vi "Mod_OFDM_Complex_Symbols _Generation.vi"(0 "Configuration in":variant, 11 "error in (no error)":errorcluster) -> (2 "Bits Generated":i8[](array[numeric]), 4 "Complex Symbols w/ Cyclic prefix":cdb[](array[numeric]), 6 "Parameters per Ofdm Symbol":T1 {"Data Source"."Data Source"."Register Initial State" format="%08x"}, 8 "Complex Symbols":cdb[][](array[numeric]), 10 "Pulse Shaping Parameters":T2={"System Filter"={"TX Filter"=enum."Root Raised Cos", "Alpha"=0.5, "filter length"=8}, "Modulation system parameters"={"samples per symbol (16)"=16}, "symbol rate (Hz)"=1.0} {"symbol rate (Hz)" min=1.0 step=1.0 format="%.2p"; "Modulation system parameters"."samples per symbol (16)" step=2; "System Filter"."Alpha" min=0.0 max=1.0 step=0.05 format="%.2f"}, 13 "Complex Mapping":cdb[][](array[numeric]), 15 "error out":errorcluster)   [LabVIEW 2010]
doc: "The VI generates the baseband complex symbols for the configured OFDM frame. Following five functions are performed by VI.l\n\n1. Converts Variant: Recovers the configuration settings from the variant into an array of clusters. The size of the array is the number of OFDM Symbols in the frame. Each cluster contains the configuration settings pertaining to a specific OFDM symbol. \n\n2. Generates Bits: For each OFDM Symbol in the Frame bits are generated depending on the data sources assigned to the sub carriers and the configuration settings of the data sources.\n\n3. Performs Complex Mapping: Complex Mapping of the bits generated are performed based on the modulation scheme selected.\n\n4. Applies IFFT: Block IFFT is performed on the complex signal\n\nNote: The common way to implement the inverse Fourier transform is by an inverse Fast Fourier Transform (IFFT). If, for example, a 64-point IFFT is used, the coefficients 0 to +31 are mapped to the same numbered IFFT inputs, while the coefficients -32 to -1 are copied into IFFT inputs +32 to +63. \n\n5. After performing an IFFT, the output is cyclically extended to the desired length by prepending the output of the IFFT."
uses:
  Controls(Type_DEf)/Configure Pulse Shaping.ctl
  Controls(Type_DEf)/Parameters per Ofdm Symbol.ctl
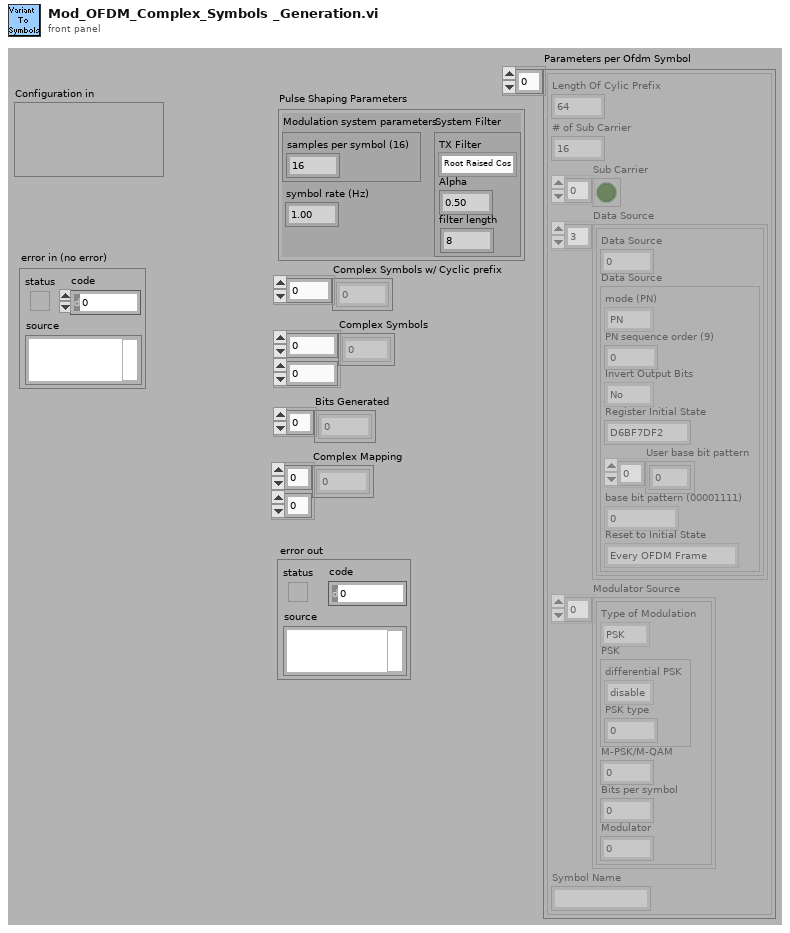
[diagram p1: front panel]
types:
  T1 = typedef "Parameters per Ofdm Symbol.ctl" = cluster{"Length Of Cylic Prefix":i32, "# of Sub Carrier":i32, "Sub Carrier":bool[], "Data Source":cluster{"Data Source":u16, "Data Source":cluster{"mode (PN)":enum16{"PN", "pattern", "user"}, "PN sequence order (9)":i32, "Invert Output Bits":enum16{"No", "Yes"}, "Register Initial State":u32, "User base bit pattern":i8[], "base bit pattern (00001111)":enum16{"0", "1", "01", "0011", "00001111"}, "Reset to Initial State":enum16{"Every OFDM Frame", "Every OFDM Symbol", "Every Sub Carrier"}}}[], "Modulator Source":cluster{"Type of Modulation":enum16{"PSK", "QAM"}, "PSK":cluster{"differential PSK":enum16{"disable", "enable"}, "PSK type":u16}, "M-PSK/M-QAM":i32, "Bits per symbol":i32, "Modulator":u16}[], "Symbol Name":string}[]
  T2 = typedef "Configure Pulse Shaping.ctl" = cluster{"System Filter":cluster{"TX Filter":enum16{"none", "Raised Cosine", "Root Raised Cos"}, "Alpha":dbl, "filter length":i32}, "Modulation system parameters":cluster{"samples per symbol (16)":u32}, "symbol rate (Hz)":dbl}
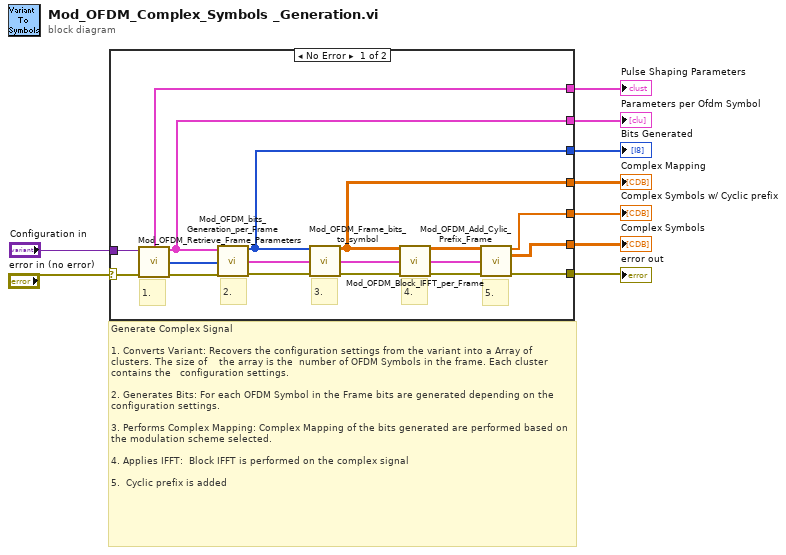
[diagram p0: block diagram]
diagram:
  # "Generate Complex Signal\n\n1. Converts Variant: Recovers the configuration settings from the variant into a Array of clusters. The size of    the array is the  number of OFDM Symbols in the frame. Each cluster contains the   configuration settings. \n\n2. Generates Bits: For each OFDM Symbol in the Frame bits are generated depending on the configuration settings.\n\n3. Performs Complex Mapping: Complex Mapping of the bits generated are performed based on the modulation scheme selected.\n\n4. Applies IFFT:  Block IFFT is performed on the complex signal\n\n5.  Cyclic prefix is added"
  n1 = case shown="No Error" "error in (no error)" {
    selector: "error in (no error)" -> [w10 w28]
    tunnel: [w24 _] -> w9
    tunnel: [w23 _] -> w8
    tunnel: "Configuration in" -> [w22 _]
    tunnel: [w21 w28] -> w6
    tunnel: [w14 _] -> w5
    tunnel: [w11 _] -> w4
    tunnel: [w15 _] -> w2
    tunnel: [w13 _] -> w1
    frame No Error {
      # "5."
      # "4."
      # "3."
      # "2."
      # "1."
      n2 = call "Mod_OFDM_Retrieve_Frame_Parameters.vi"("Configuration in"=w22, "error in (no error)"=w10) -> ("Pulse Shaping Parameters"=w14:T2, "Parameters per Ofdm Symbol"=w15:T1, "Initial SEED IN"=w12:u32[], "error out"=w16:errorcluster)  [unwired: 10 in]
      n3 = call "Mod_OFDM_bits_Generation_per_Frame.vi"("Parameters per Ofdm Symbol"=w15, "Initial SEED IN"=w12, "error in (no error)"=w16) -> ("Bits Generated"=w11:i8[], "Parameters per Ofdm Symbol"=w20:T1, "error out"=w27:errorcluster)  [unwired: 10 in]
      n4 = call "Mod_OFDM_Frame_bits_to_symbol.vi"("Bits Generated"=w11, "Parameters per Ofdm Symbol"=w20, "error in"=w27) -> ("Complex Mapping"=w13:cdb[][], "Parameters per Ofdm Symbol"=w19:T1, "error out"=w26:errorcluster)  [unwired: 10 in]
      n5 = call "Mod_OFDM_Block_IFFT_per_Frame.vi"("Complex Mapping"=w13, "Parameters per Ofdm Symbol"=w19, "error in (no error)"=w26) -> ("IFFT Out"=w17:cdb[][], "Parameters per Ofdm Symbol"=w18:T1, "error out"=w25:errorcluster)  [unwired: 10 in]
      n6 = call "Mod_OFDM_Add_Cylic_Prefix_Frame.vi"("Complex IFFT"=w17, "Parameters per Ofdm Symbol"=w18, "error in"=w25) -> ("Complex Symbols w/  Cyclic prefix"=w24:cdb[], "Complex IFFT w/ Cyclic Prefix"=w23:cdb[][], "error out"=w21:errorcluster)  [unwired: 10 in]
    }
    frame Error {
    }
  }
  "Complex Symbols w/ Cyclic prefix" <- w9
  "Complex Symbols" <- w8
  "error out" <- w6
  "Pulse Shaping Parameters" <- w5
  "Bits Generated" <- w4
  "Parameters per Ofdm Symbol" <- w2
  "Complex Mapping" <- w1
